vi "instr.Serial.FrameReader.vi"(0 "VISA resource name":refnum<visa-resource-name> caption="Serial Port", 1 "timeout (10sec)":u32=1000 caption="TimeOut", 5 "baud rate (9600)":u32=9600 caption="BaudRate(9600)", 7 "Send Mode":T1(ring), 9 "Send":string, 11 "error in (no error)":errorcluster caption="错误输入（无错误）", 12 "Return Length":u32) -> (4 "ok?":bool, 6 "Return":string, 15 "error out":errorcluster caption="错误输出")   [LabVIEW 2012, in "Lib_UEL.ATE.lvlib" / "Lib_Instrument.lvlib"]
uses:
  Lib_Instrument.lvlib
  <vilib>/Instr/_visa.llb/VISA Configure Serial Port (Instr).vi
  App/Lib_App.lvlib
panel:
  # "V1.0 - Replace old frame WR.~LI.Guang 2015-5-8"
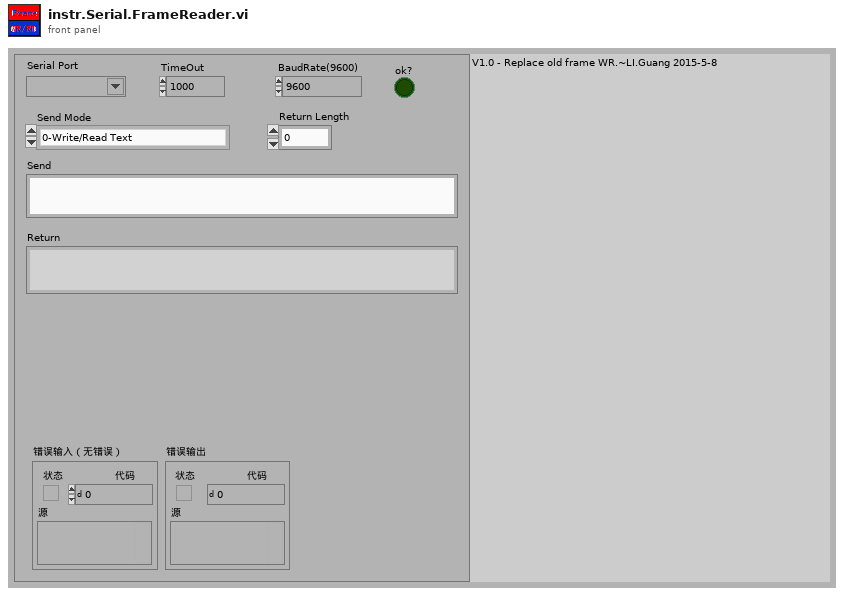
[diagram p1: front panel]
types:
  T1 = enum16{"0-Write/Read Text", "1-Write/Read Hex", "2-Read ONLY(Hex)"}
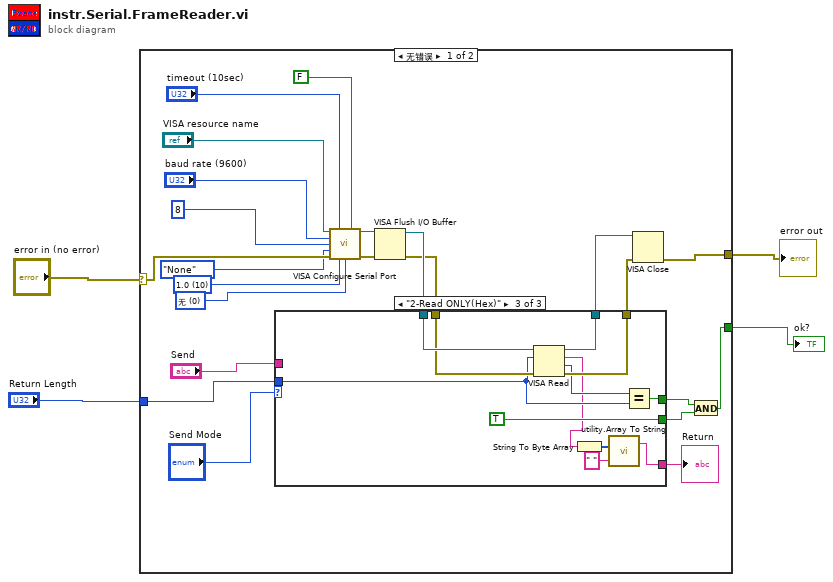
[diagram p0: block diagram]
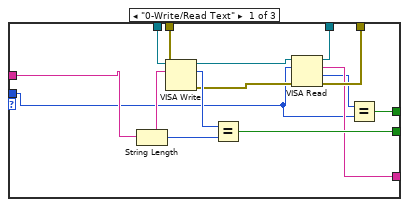
[diagram p2: hidden frame]
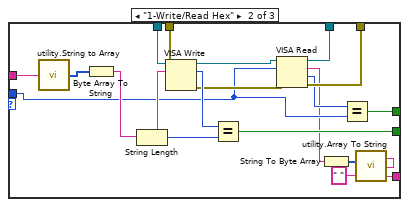
[diagram p3: hidden frame]
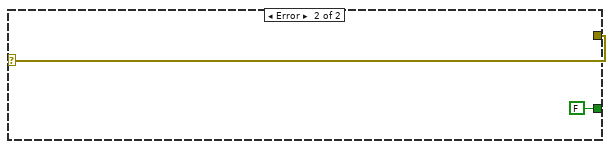
[diagram p4: hidden frame]
diagram:
  n1 = case shown="无错误" "error in (no error)" {
    selector: "error in (no error)" -> [w24 w74]
    tunnel: [w23 w74] -> w3
    tunnel: "Return Length" -> [w9 _]
    tunnel: [w12 FALSE] -> w1
    frame No Error {
      w17 = u16 0 items=["无", "XON/XOFF", "RTS/CTS", "XON/XOFF & RTS/CTS", "DTR/DSR", "XON/XOFF & DTR/DSR"] ("flow control (0:none)")
      w18 = u16 10 items=["1.0"=10, "1.5"=15, "2.0"=20] ("stop bits (10: 1 bit)")
      n2 = call-poly "VISA Configure Serial Port"("VISA resource name"="VISA resource name", "timeout (10sec)"="timeout (10sec)", "Enable Termination\nChar (T)"=FALSE ("Disable Termination\nChar (T)"), "baud rate (9600)"="baud rate (9600)", "data bits (8)"=u16 8, "parity (0:none)"=enum16{"None", "Odd", "Even", "Mark", "Space"}."None", "error in (no error)"=w24, "stop bits (10: 1 bit)"=w18, "flow control (0:none)"=w17) -> ("VISA resource name out"=w15:refnum<visa-resource-name>, "error out"=w16:errorcluster)  [unwired: 5 in]
      n3 = VISA Flush I/O Buffer(VISA resource name=w15, error in (no error)=w16) -> (VISA resource name out=w14:refnum<visa-resource-name>, error out=w13:errorcluster)  [unwired: 1 in]
      n4 = case shown="\"2-Read ONLY(Hex)\"" "Send Mode" {
        tunnel: [w39 w58 TRUE] -> w22
        tunnel: w14 -> [w38 w57 w71]
        tunnel: w13 -> [w37 w56 w70]
        tunnel: "Send" -> [w36 w55 _]
        tunnel: w9 -> [w29 w47 w65]
        tunnel: [w33 w50 w69] -> w8
        tunnel: [w32 w49 w68] -> w7
        tunnel: [w31 w43 w61] -> w6
        tunnel: [w28 w46 w67] -> w5
        frame "0-Write/Read Text" {
          n5 = String Length(string=w36) -> (length=w41:i32)
          n6 = VISA Write(VISA resource name=w38, write buffer=w36, error in (no error)=w37) -> (VISA resource name out=w35:refnum<visa-resource-name>, return count=w40:u32, error out=w34:errorcluster)
          n7 = Equal?(x=w40, y=w41) -> (x = y?=w39:bool)
          n8 = VISA Read(VISA resource name=w35, byte count=w29, error in (no error)=w34) -> (VISA resource name out=w33:refnum<visa-resource-name>, read buffer=w31:string, return count=w30:u32, error out=w32:errorcluster)
          n9 = Equal?(x=w30, y=w29) -> (x = y?=w28:bool)
        }
        frame "1-Write/Read Hex" {
          n10 = call "utility.String to Array.vi"("命令输入"=w55) -> ("输出数组"=w54:u8[])
          n11 = Byte Array To String(unsigned byte array=w54) -> (string=w53:string)
          n12 = String Length(string=w53) -> (length=w60:i32)
          n13 = VISA Write(VISA resource name=w57, write buffer=w53, error in (no error)=w56) -> (VISA resource name out=w52:refnum<visa-resource-name>, return count=w59:u32, error out=w51:errorcluster)
          n14 = Equal?(x=w59, y=w60) -> (x = y?=w58:bool)
          n15 = VISA Read(VISA resource name=w52, byte count=w47, error in (no error)=w51) -> (VISA resource name out=w50:refnum<visa-resource-name>, read buffer=w45:string, return count=w48:u32, error out=w49:errorcluster)
          n16 = String To Byte Array(string=w45) -> (unsigned byte array=w44:u8[])
          n17 = Equal?(x=w48, y=w47) -> (x = y?=w46:bool)
          n18 = call "utility.Array To String.vi"("分隔符输入"=" ", "无符号字节数组"=w44) -> ("命令输出(字符串)"=w43:string)  [unwired: 1 out]
        }
        frame "2-Read ONLY(Hex)" {
          n19 = VISA Read(VISA resource name=w71, byte count=w65, error in (no error)=w70) -> (VISA resource name out=w69:refnum<visa-resource-name>, read buffer=w62:string, return count=w66:u32, error out=w68:errorcluster)
          n20 = String To Byte Array(string=w62) -> (unsigned byte array=w64:u8[])
          n21 = call "utility.Array To String.vi"("分隔符输入"=" ", "无符号字节数组"=w64) -> ("命令输出(字符串)"=w61:string)  [unwired: 1 out]
          n22 = Equal?(x=w66, y=w65) -> (x = y?=w67:bool)
        }
      }
      "Return" <- w6
      n23 = VISA Close(VISA resource name=w8, error in (no error)=w7) -> (error out=w23:errorcluster)
      n24 = And(x=w5, y=w22) -> (x .and. y?=w12:bool)
    }
    frame Error {
    }
  }
  "error out" <- w3
  "ok?" <- w1
